vi "Append Watermark Text.vi"(0 "PDF Report IN":refnum<class "PDF Report Class.lvclass">, 2 "Watermark Text":T1={"Text "="CONFIDENTIAL", "Opacity (%)"=10.0, "Position"={"Position"=enum."Center (text section)", "X"=0.0, "Y"=0.0}, "Automatic"=FALSE, "Font"={"Font Name"="", "Size"=-1.0, "Color"=0}, "Alignment"=enum."Left", "Rotate(°)"=0.0}, 11 "error in (no error)":errorcluster) -> (4 "PDF Report OUT":refnum<class "PDF Report Class.lvclass">, 15 "error out":errorcluster)   [LabVIEW 2020, in "Exaprom PDF.lvlib"]
doc: "Appends a <B>watermark</B> (text or image) on each page of the PDF report. \n\n<B>FRANÇAIS</B>\nAjoute un <B>filigrane</B> (texte or image) sur chaque page du rapport PDF. \n\nVersion 1.0\nDeveloped by Jean-Marc Simard\nCopyright © 2010, Exaprom Inc.\nAll rights reserved.\nLicense: BSD\n\nWith iTextSharp Library\n(http://itextsharp.sourceforge.net)"
uses:
  <userlib>/labview-PDF-writer-master/Exaprom PDF.lvlib
  <userlib>/labview-PDF-writer-master/LV Class/PDF Report Class/PDF Report Class.lvclass
  <userlib>/labview-PDF-writer-master/Controls/Header, Footer and Watermark Controls/Watermark Text Cluster.ctl
  <userlib>/labview-PDF-writer-master/Controls/Header, Footer and Watermark Controls/Watermark Position.ctl
  <userlib>/labview-PDF-writer-master/Controls/Font Controls/Font size.ctl
  <userlib>/labview-PDF-writer-master/Controls/Font Controls/Font color.ctl
  <userlib>/labview-PDF-writer-master/Controls/Header, Footer and Watermark Controls/Header footer horiz alignment.ctl
  <userlib>/labview-PDF-writer-master/Controls/Font Controls/Font complete cluster.ctl
  <userlib>/labview-PDF-writer-master/Controls/Font Controls/Type and encoding.ctl
  <userlib>/labview-PDF-writer-master/Controls/Text Controls/Unicode/Type and run direction.ctl
  <userlib>/labview-PDF-writer-master/LV Class/Fonts Class/Font Class.lvclass
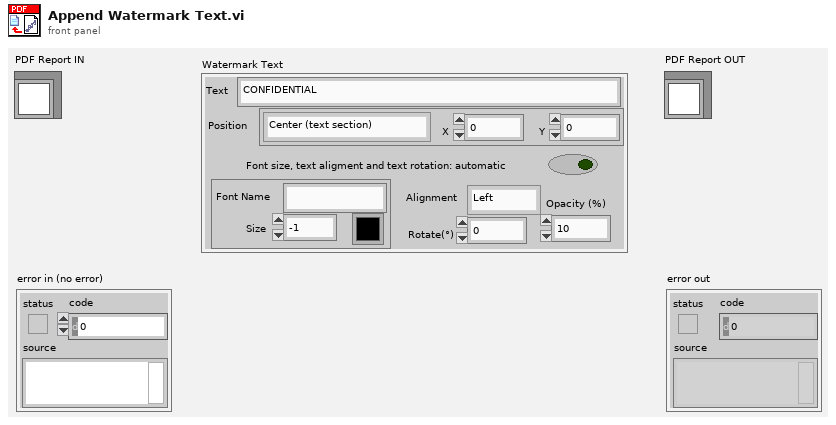
[diagram p1: front panel]
types:
  T1 = typedef "Exaprom PDF.lvlib/Watermark Text Cluster.ctl" = cluster{"Text ":string, "Opacity (%)":sgl, "Position":cluster{"Position":T2, "X":sgl, "Y":sgl}, "Automatic":bool, "Font":cluster{"Font Name":string, "Size":T3, "Color":T4}, "Alignment":T5, "Rotate(°)":sgl}
  T2 = typedef "Exaprom PDF.lvlib/Watermark Position.ctl" = enum16{"Absolute", "Center (page)", "Center (text section)"}
  T3 = typedef "Exaprom PDF.lvlib/Font size.ctl" = sgl
  T4 = typedef "Exaprom PDF.lvlib/Font color.ctl" = u32
  T5 = typedef "Exaprom PDF.lvlib/Header footer horiz alignment.ctl" = enum16{"Left", "Center", "Right"}
  T6 = typedef "Exaprom PDF.lvlib/Font complete cluster.ctl" = cluster{"Name":string, "Size":T3, "Color":T4, "Style":cluster{"Bold":bool, "Italic":bool, "Underline":bool, "Strikeout":bool}, "Type":T7}
  T7 = typedef "Exaprom PDF.lvlib/Type and encoding.ctl" = cluster{"Type&direction":T8, "Embedded":bool, "Encoding":string}
  T8 = typedef "Exaprom PDF.lvlib/Type and run direction.ctl" = enum16{"Select", "ASCII", "UTF-16", "UTF-16 (default)", "UTF-16 (LTR)", "UTF-16 (RTL)"}
  T9 = typedef "Exaprom PDF.lvlib/Watermark cluster2.ctl" = cluster{"Show? (F)":bool, "Type":enum16{"Image", "Text"}, "Opacity (%)":sgl, "Rotate(°)":sgl, "Position":cluster{"Position":T2, "X":sgl, "Y":sgl}, "Image path":path, "Scaled(%)":sgl, "Image refnum":refnum<k24>, "Text":string, "Font":cluster{"Name":string, "Size":T3, "Color":T4}, "Font refnum":refnum<k24>, "Alignment":T5, "Automatic":bool}
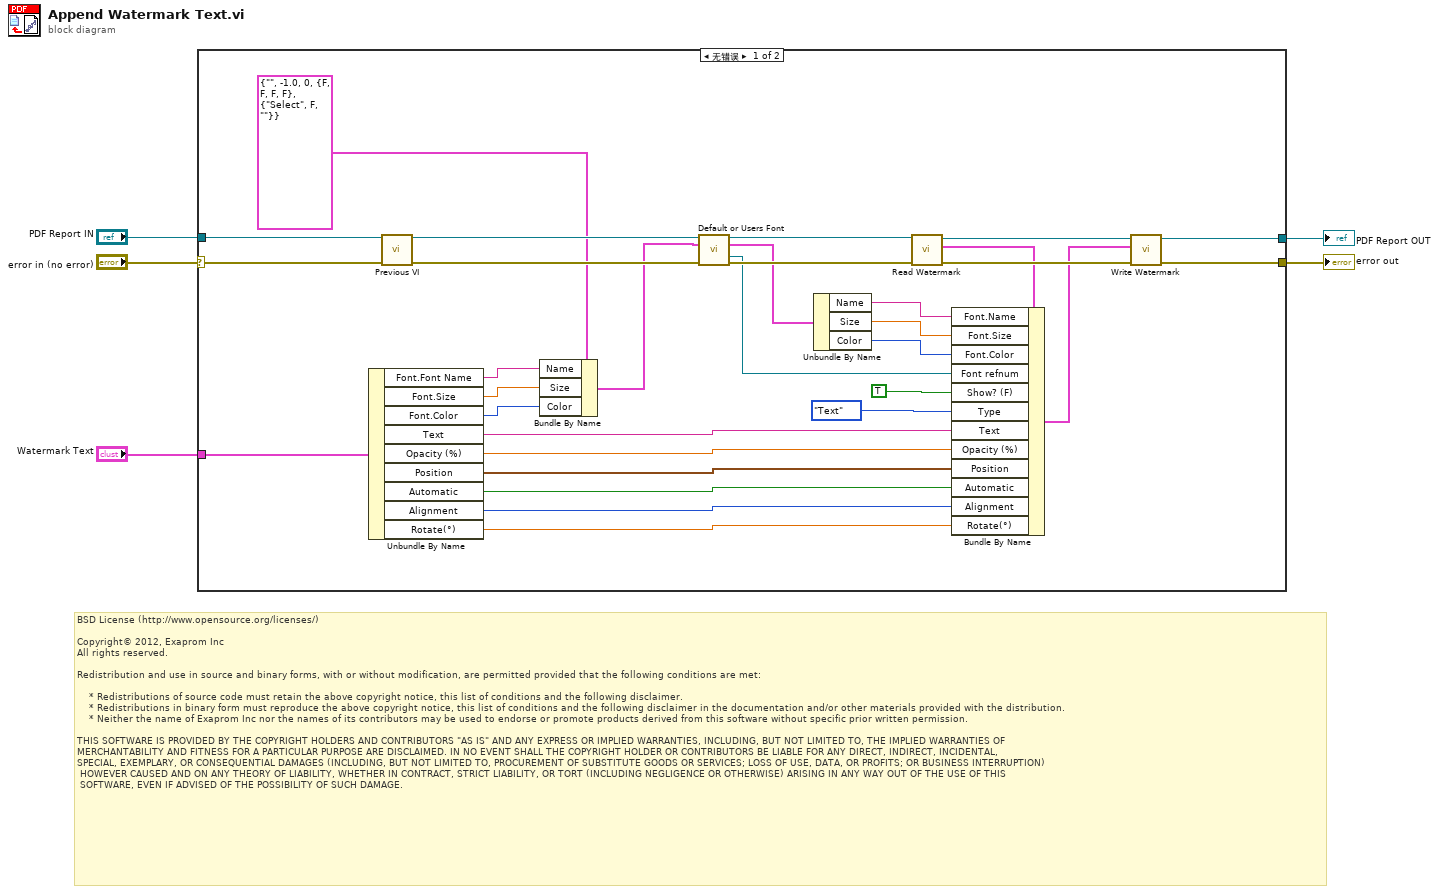
[diagram p0: block diagram]
diagram:
  # "BSD License (http://www.opensource.org/licenses/)\n\nCopyright© 2012, Exaprom Inc\nAll rights reserved.\n\nRedistribution and use in source and binary forms, with or without modification, are permitted provided that the following conditions are met:\n\n    * Redistributions of source code must retain the above copyright notice, this list of conditions and the following disclaimer.\n    * Redistributions in binary form must reproduce the above copyright notice, this list of conditions and the following disclaimer in the documentation and/or other materials provided with the distribution.\n    * Neither the name of Exaprom Inc nor the names of its contributors may be used to endorse or promote products derived from this software without specific prior written permission.\n\nTHIS SOFTWARE IS PROVIDED BY THE COPYRIGHT HOLDERS AND CONTRIBUTORS \"AS IS\" AND ANY EXPRESS OR IMPLIED WARRANTIES, INCLUDING, BUT NOT LIMITED TO, THE IMPLIED WARRANTIES OF \nMERCHANTABILITY AND FITNESS FOR A PARTICULAR PURPOSE ARE DISCLAIMED. IN NO EVENT SHALL THE COPYRIGHT HOLDER OR CONTRIBUTORS BE LIABLE FOR ANY DIRECT, INDIRECT, INCIDENTAL,\nSPECIAL, EXEMPLARY, OR CONSEQUENTIAL DAMAGES (INCLUDING, BUT NOT LIMITED TO, PROCUREMENT OF SUBSTITUTE GOODS OR SERVICES; LOSS OF USE, DATA, OR PROFITS; OR BUSINESS INTERRUPTION)\n HOWEVER CAUSED AND ON ANY THEORY OF LIABILITY, WHETHER IN CONTRACT, STRICT LIABILITY, OR TORT (INCLUDING NEGLIGENCE OR OTHERWISE) ARISING IN ANY WAY OUT OF THE USE OF THIS\n SOFTWARE, EVEN IF ADVISED OF THE POSSIBILITY OF SUCH DAMAGE."
  n1 = case shown="无错误" "error in (no error)" {
    selector: "error in (no error)" -> [w34 w38]
    tunnel: "PDF Report IN" -> [w35 w37]
    tunnel: "Watermark Text" -> [w33 _]
    tunnel: [w8 w37] -> w3
    tunnel: [w11 w38] -> w2
    frame No Error {
      n2 = Unbundle By Name(w33) -> ("Font.Font Name"=w22:string, "Font.Size"=w21:T3, "Font.Color"=w20:T4, "Text"=w30:string, "Opacity (%)"=w29:sgl, "Position"=w28:cluster{"Position":T2, "X":sgl, "Y":sgl}, "Automatic"=w27:bool, "Alignment"=w26:T5, "Rotate(°)"=w25:sgl)
      n3 = call <userlib>:"Previous VI.vi"("PDF Report IN"=w35, "error in (no error)"=w34) -> ("PDF Report OUT"=w24:refnum<class "PDF Report Class.lvclass">, "error out"=w23:errorcluster)  [unwired: 12 out]
      n4 = Bundle By Name(cluster=T6 {"Name"="", "Size"=-1.0, "Color"=0, "Style"={"Bold"=FALSE, "Italic"=FALSE, "Underline"=FALSE, "Strikeout"=FALSE}, "Type"={"Type&direction"=enum."Select", "Embedded"=FALSE, "Encoding"=""}} ("Font"), "Name"=w22, "Size"=w21, "Color"=w20) -> (w6:T6)
      n5 = call <userlib>:"Default or Users Font.vi"("PDF Report"=w24, "Font"=w6, "error in (no error)"=w23) -> ("PDF Report duplicate"=w13:refnum<class "PDF Report Class.lvclass">, "Font OUT"=w19:T6, "Font Ref"=w15:refnum<k24>, "error out"=w36:errorcluster)  [unwired: 7 in, 2 out]
      n6 = Unbundle By Name(w19) -> ("Name"=w18:string, "Size"=w17:T3, "Color"=w16:T4)
      n7 = call-dynamic "Read Watermark .vi"("error in (no error)"=w36, "PDF Report Class in"=w13) -> ("error out"=w14:errorcluster, "Watermark Cluster"=w12:T9, "PDF Report Class out"=w9:refnum<class "PDF Report Class.lvclass">)  [unwired: 7 in]
      n8 = Bundle By Name(cluster=w12, "Font.Name"=w18, "Font.Size"=w17, "Font.Color"=w16, "Font refnum"=w15, "Show? (F)"=TRUE ("Watermark .Show? (F)"), "Type"=enum16{"Image", "Text"}."Text" ("Watermark .Type"), "Text"=w30, "Opacity (%)"=w29, "Position"=w28, "Automatic"=w27, "Alignment"=w26, "Rotate(°)"=w25) -> (w10:T9)
      n9 = call-dynamic "Write Watermark .vi"("error in (no error)"=w14, "Watermark Cluster"=w10, "PDF Report Class in"=w9) -> ("error out"=w11:errorcluster, "PDF Report Class out"=w8:refnum<class "PDF Report Class.lvclass">)  [unwired: 7 in]
    }
    frame Error {
    }
  }
  "PDF Report OUT" <- w3
  "error out" <- w2
